vi "Create Line.vi"(8 "error in (no error)":errorcluster) -> (0 "error out":errorcluster, 3 "Line out":refnum<class "Line.lvclass">)   [LabVIEW 2015, in "LV Image Editor Framework.lvlib" / "Line.lvclass"]
uses:
  Line.lvclass
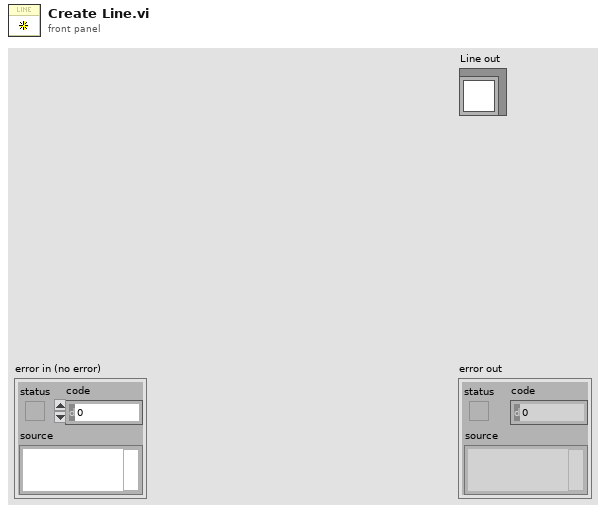
[diagram p1: front panel]
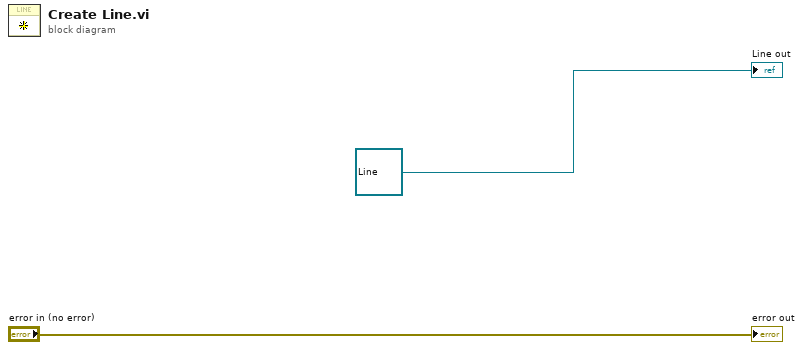
[diagram p0: block diagram]
diagram:
  "error out" <- "error in (no error)"
  "Line out" <- refnum<class "Line.lvclass"> refnum ("Line in")
